vi "实验报表路径.vi"() -> ()   [LabVIEW 2013]
panel:
  in  "实验报表路径":path=path "D:/研究生/课程/油动机项目/实验文件夹/DR96-03-5/GV1/GV1-表格.txt"
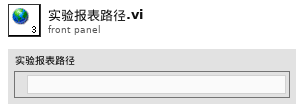
[diagram p1: front panel]
diagram:
